vi "Wrap2Wind Demo.vi"() -> ()   [LabVIEW 2016]
uses:
  <vilib>/addons/control/pid/pid.llb/PID Output Rate Limiter (DBL).vi
  <vilib>/addons/control/pid/NI_PID_pid.lvlib
panel:
  in  "Behavior":bool
  out "In 3":dbl=9.29032258064521
  out "x-y":dbl=9.29032258064521
  out "Out 2":dbl=9.29032258064521
  out "Out":dbl(slide)=9.29032258064521 scale=-720.0..720.0
  out "In 2":dbl(slide)=9.29032258064521 scale=-720.0..720.0
  in  "output rate (EGU/min)":dbl=1000000.0 format="%.2f"
  in  "In":dbl(slide)=4.884981308350689e-14 scale=-720.0..720.0
  # "Robot Physical Yaw"
  # "What Wrapped Sensor Reports"
  # "F: 0-360\nT: +/-180"
  # "Reported after Wrap2Wind Treatment"
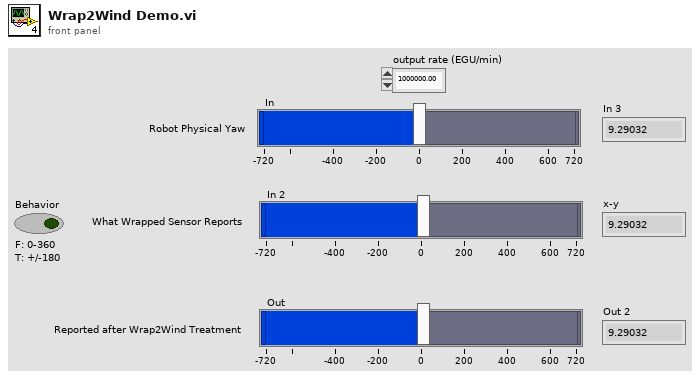
[diagram p1: front panel]
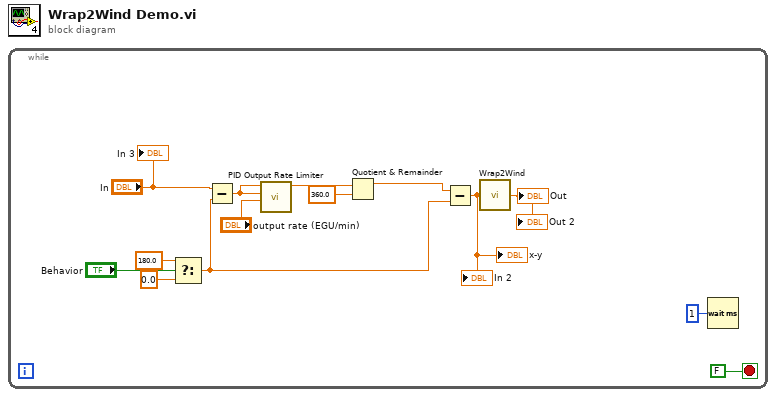
[diagram p0: block diagram]
diagram:
  n1 = while {
    stop <- FALSE stop-if-true
    n2 = Select(t=180.0 ("y"), s="Behavior", f=0.0) -> (s? t:f=w2:dbl)
    n3 = Subtract(x="In", y=w2) -> (x-y=w5:dbl)
    n4 = call-poly <vilib>:"PID Output Rate Limiter.vi"("output rate (EGU/min)"="output rate (EGU/min)", "initial output"=w5, "input (controller output)"=w5) -> ("output"=w11:dbl)  [unwired: 5 in, 1 out]
    n5 = Quotient & Remainder(x=w11, y=360.0) -> (x-y*floor(x/y)=w8:dbl)  [unwired: 1 out]
    n6 = Subtract(x=w8, y=w2) -> (x-y=w7:dbl)
    "In 2" <- w7
    "x-y" <- w7
    n7 = call "Wrap2Wind.vi"("In"=w7) -> ("Out"=→"Out" →"Out 2":dbl)  [unwired: 4 in]
    n8 = Wait (ms)(milliseconds to wait=u32 1) -> ()  [unwired: 1 out]
    "In 3" <- "In"
  }
